vi "Inst.TSL210.DoSomething.vi"(8 "error in (no error)":errorcluster, 10 "Data":variant, 11 "Inst.TSL210 in":refnum<class "Inst.TSL210.lvclass">) -> (0 "error out":errorcluster, 2 "Data out":variant, 3 "Inst.TSL210 out":refnum<class "Inst.TSL210.lvclass">)   [LabVIEW 2019, in "Inst.TSL210.lvclass"]
uses:
  Inst.TSL210.lvclass
  fdab1b40-c942-4d42-9f74-5965e28da6e4.vi
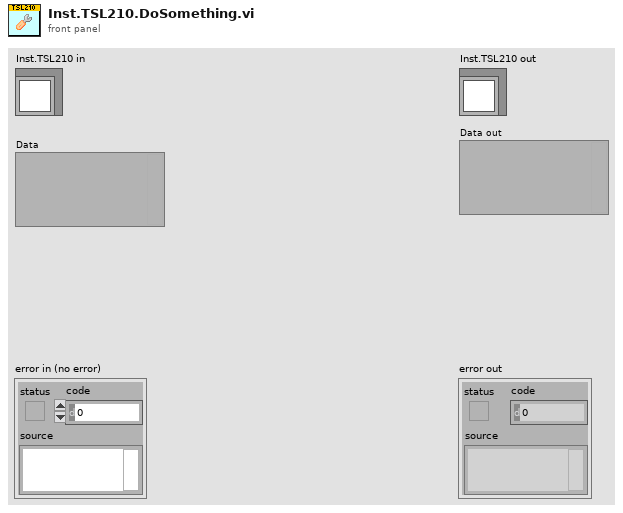
[diagram p1: front panel]
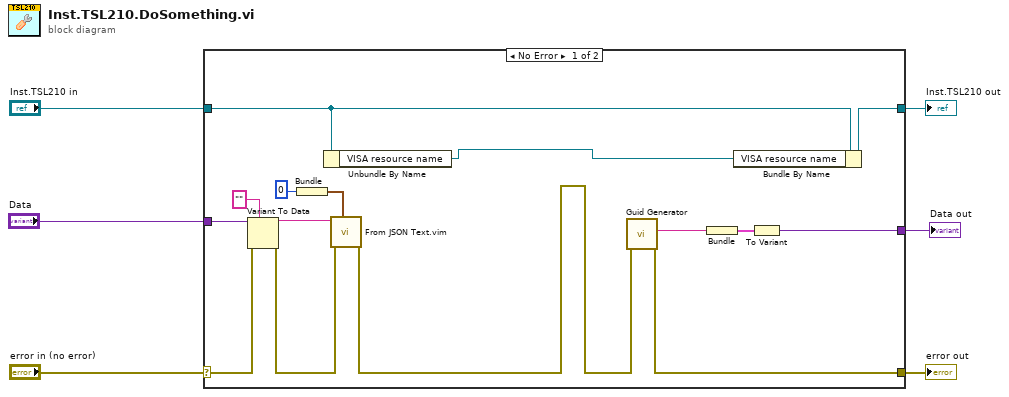
[diagram p0: block diagram]
diagram:
  n1 = case shown="No Error" "error in (no error)" {
    selector: "error in (no error)" -> [w17 w23]
    tunnel: [w11 w23] -> w5
    tunnel: [w21 w22] -> w3
    tunnel: "Inst.TSL210 in" -> [w20 w22]
    tunnel: "Data" -> [w19 _]
    tunnel: [w10 _] -> w1
    frame No Error {
      n2 = Variant To Data(error in=w17, type="", Variant=w19) -> (data=w16:string, error out=w15:errorcluster)
      n3 = Bundle("bytes to read"=0) -> (w14:cluster{"bytes to read":i32})  [unwired: 1 in]
      n4 = Unbundle By Name(w20) -> ("VISA resource name"=w8:refnum<visa-resource-name>)
      n5 = call "From JSON Text.vim"("Data Type and Default Value"=w14, "error in (no error)"=w15, "JSON"=w16) -> ("error out"=w7:errorcluster)  [unwired: 7 in, 1 out]
      n6 = call <vilib>:"Guid Generator.vi"("error in (no error)"=w7) -> ("error out"=w11:errorcluster, "GUID"=w12:string)  [unwired: 9 in]
      n7 = Bundle("GUID"=w12) -> (w9:cluster{"GUID":string})  [unwired: 1 in]
      n8 = Bundle By Name(cluster=w20, "VISA resource name"=w8) -> (w21:refnum<class "Inst.TSL210.lvclass">)
      n9 = To Variant(anything=w9) -> (Variant=w10:variant)
    }
    frame Error {
    }
  }
  "error out" <- w5
  "Inst.TSL210 out" <- w3
  "Data out" <- w1
